vi "ImageFormatConvert.vi"(0 "pInputBuffer":u8[](array[numeric]), 1 "nWidth":u32, 2 "nHeight":u32, 3 "nSrcPixelFormat":i32, 4 "nDstPixelFormat":i32, 5 "nValidBits":i32, 6 "bFlip":bool=TRUE, 7 "error in (no error)":errorcluster, 9 "nConvertType":i32) -> (21 "nOutputBuffer":u8[](array[numeric]), 23 "nOutPutBufferSize":i64, 27 "error out":errorcluster)   [LabVIEW 2016, in "GxLVLib.lvlib"]
uses:
  GxLVLib.lvlib
  DxImageProc.dll
panel:
  out "DX_STATUS 8":i32
  in  "DX_STATUS 7":i32
  out "DX_STATUS 6":i32
  out "DX_STATUS 5":i32
  out "DX_STATUS 4":i32
  in  "DX_STATUS 3":i32
  out "DX_STATUS 2":i32
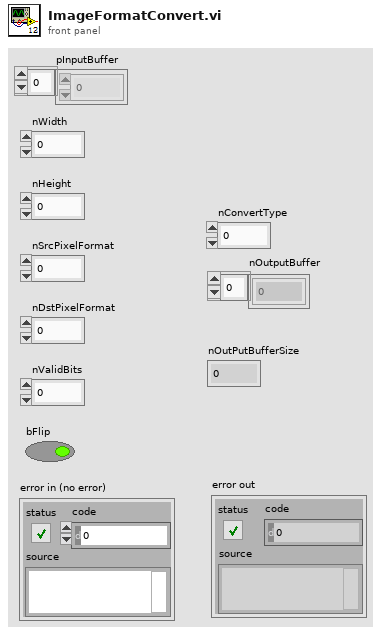
[diagram p1: front panel]
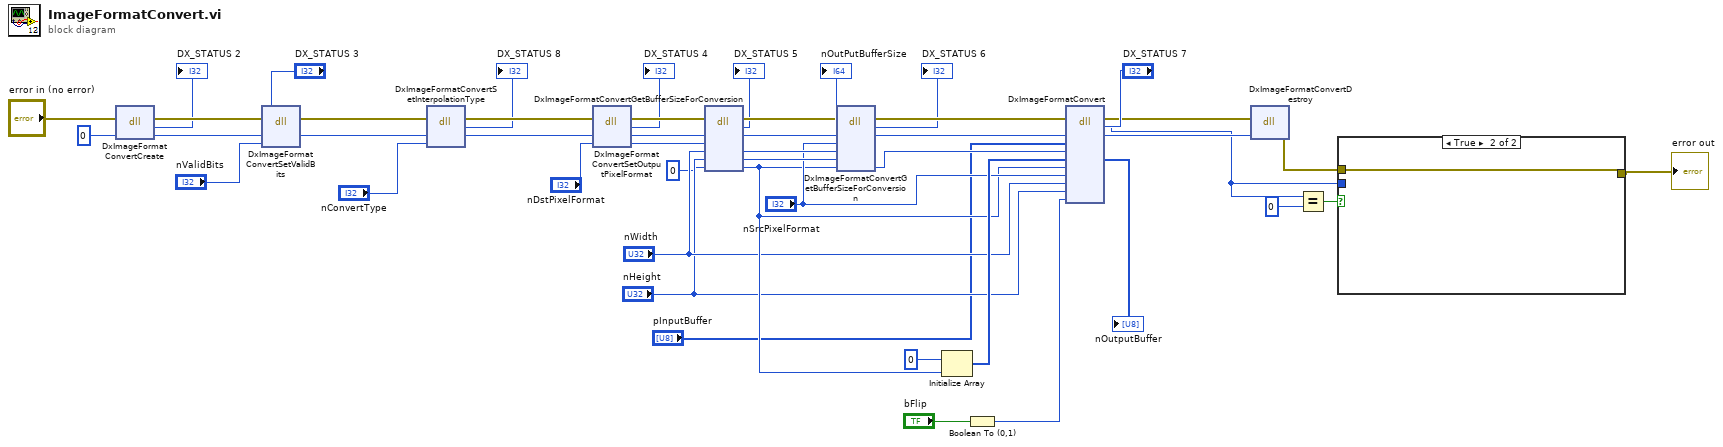
[diagram p0: block diagram]
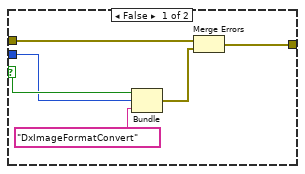
[diagram p2: hidden frame]
diagram:
  n1 = dll-call lib="DxImageProc.dll" fn="DxImageFormatConvertCreate"(error in="error in (no error)", "handle"=0) -> (error out=w39:errorcluster, "DX_STATUS"=→"DX_STATUS 2":i32, "handle"=w46:i64)  [unwired: 2 in, 1 out]
  n2 = dll-call lib="DxImageProc.dll" fn="DxImageFormatConvertSetValidBits"(error in=w39, "DX_STATUS"="DX_STATUS 3", "handle"=w46, "emValidBits"="nValidBits") -> (error out=w10:errorcluster, "handle"=w7:i64)  [unwired: 3 in, 1 out]
  n3 = dll-call lib="DxImageProc.dll" fn="DxImageFormatConvertSetInterpolationType"(error in=w10, "handle"=w7, "emConvertType"="nConvertType") -> (error out=w9:errorcluster, "DX_STATUS"=→"DX_STATUS 8":i32, "handle"=w6:i64)  [unwired: 3 in, 1 out]
  n4 = dll-call lib="DxImageProc.dll" fn="DxImageFormatConvertSetOutputPixelFormat"(error in=w9, "handle"=w6, "emPixelFormat"="nDstPixelFormat") -> (error out=w20:errorcluster, "DX_STATUS"=→"DX_STATUS 4":i32, "handle"=w32:i64, "emPixelFormat"=w31:i32)  [unwired: 2 in, 1 out]
  n5 = dll-call lib="DxImageProc.dll" fn="DxImageFormatConvertGetBufferSizeForConversion"(error in=w20, "handle"=w32, "emPixelFormat"=w31, "nImgWidth"="nWidth", "nImgHeight"="nHeight", "pBufferSize"=i64 0) -> (error out=w19:errorcluster, "DX_STATUS"=→"DX_STATUS 5":i32, "handle"=w30:i64, "nImgWidth"=w29:u32, "nImgHeight"=w28:u32, "pBufferSize"=w24:i32)  [unwired: 3 in, 1 out]
  "nOutPutBufferSize" <- w24
  n6 = dll-call lib="DxImageProc.dll" fn="DxImageFormatConvertGetBufferSizeForConversion"(error in=w19, "handle"=w30, "emPixelFormat"="nSrcPixelFormat", "nImgWidth"=w29, "nImgHeight"=w28) -> (error out=w18:errorcluster, "DX_STATUS"=→"DX_STATUS 6":i32, "handle"=w27:i64, "pBufferSize"=w26:i32)  [unwired: 6 in, 1 out]
  n7 = Initialize Array(u8 0, w24) -> (w42:u8[])
  n8 = Boolean To (0,1)(Boolean="bFlip") -> (0, 1=w34:i16)
  n9 = dll-call lib="DxImageProc.dll" fn="DxImageFormatConvert"(error in=w18, "DX_STATUS"="DX_STATUS 7", "handle"=w27, "pInputBuffer"="pInputBuffer", "nInBufferSize"=w26, "pOutputBuffer"=w42, "nOutBufferSize"=w24, "emInPixelFormat"="nSrcPixelFormat", "nImgWidth"="nWidth", "nImgHeight"="nHeight", "bFlip"=w34) -> (error out=w4:errorcluster, "DX_STATUS"=w1:i32, "handle"=w2:i64, "pOutputBuffer"=→"nOutputBuffer":u8[])  [unwired: 8 in, 1 out]
  n10 = dll-call lib="DxImageProc.dll" fn="DxImageFormatConvertDestroy" ("DxImageFormatConvertCreate")(error in=w4, "handle"=w2) -> (error out=w3:errorcluster)  [unwired: 4 in, 1 out]
  n11 = Equal?(x=w1, y=0) -> (x = y?=w36:bool)
  n12 = case shown="True" w36 {
    selector: w36 -> [w49 _]
    tunnel: w3 -> [w52 w53]
    tunnel: [w51 w53] -> w38
    tunnel: w1 -> [w48 _]
    frame False {
      n13 = Bundle(w49, "DX_STATUS"=w48, "DxImageFormatConvert") -> (w50:cluster{bool, "DX_STATUS":i32, string})  [unwired: 1 in]
      n14 = Merge Errors(w52, w50) -> (w51:errorcluster)
    }
    frame True {
    }
  }
  "error out" <- w38
